vi "Format Attribute Value String.vi"(8 "error in (no error)":errorcluster, 11 "Data":variant) -> (0 "error out":errorcluster, 3 "Value as String":string)   [LabVIEW 2020, in "Linked Lists.lvlib" / "Linked List.lvclass"]
uses:
  <vilib>/gpm_packages/@cs/linked-list/Source/Linked List/Linked List/Linked List.lvclass
  <vilib>/gpm_packages/@cs/data-type-serializer/source/Data Type/Data Type.lvclass
  <vilib>/Utility/Data Type/NI_Data Type.lvlib
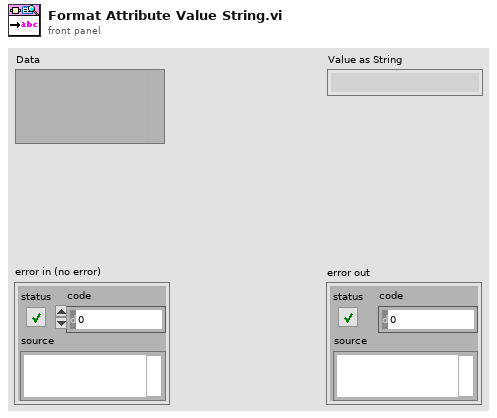
[diagram p1: front panel]
types:
  T1 = typedef "NI_Data Type.lvlib/Data Type.ctl" = enum8{"Invalid Type", "Void", "I8", "I16", "I32", "I64", "U8", "U16", "U32", "U64", "Single Float", "Double Float", "Extended Float", "Single Complex", "Double Complex", "Extended Complex", "Enum U8", "Enum U16", "Enum U32", "Enum U64", "Single Float With Unit", "Double Float With Unit", "Extended Float With Unit", "Single Complex with Unit", "Double Complex with Unit", "Extended Complex with Unit", "Boolean", "String", "Path", "Picture", "Tag", "Array", "Cluster", "Variant", "LV Variant", "Waveform", "Timestamp", "Digital Waveform", "Digital Data", "ExpressData", "Refnum", "External Data", "VI", "Poly VI", "LabVIEW Class Instance", "Fixed Point", "Set Collection", "Map Collection"}
  T2 = typedef "NI_Data Type.lvlib/Memory Info.ctl" = cluster{"Type":T3, "Size":u32}
  T3 = typedef "NI_Data Type.lvlib/Memory Type.ctl" = enum16{"Variable", "Fixed", "Bounded"}
  T4 = typedef "NI_Data Type.lvlib/Refnum Type.ctl" = enum16{"NotARefnum", "UnknownRefnum", "Generic", "Datalog", "ByteStream", "Device", "Occurence", "TCPNetConnection", "Auto", "Menu", "Imaq", "Hardware", "DataSocket", "Visa", "IVI", "UDPNetConnection", "Notifier", "Queue", "Irda", "EventReg", "DotNet", "UserEvent", "Callback", "UNUSED_EMPTY_POSITION", "BlueToothNetConnection", "LVObjApp", "LVObjVI", "LVObjUnknown", "GenericClass", "UserDefinedRefnumTag", "DataValue", "RT FIFO", "TDMS File", "PythonSessionRefnum"}
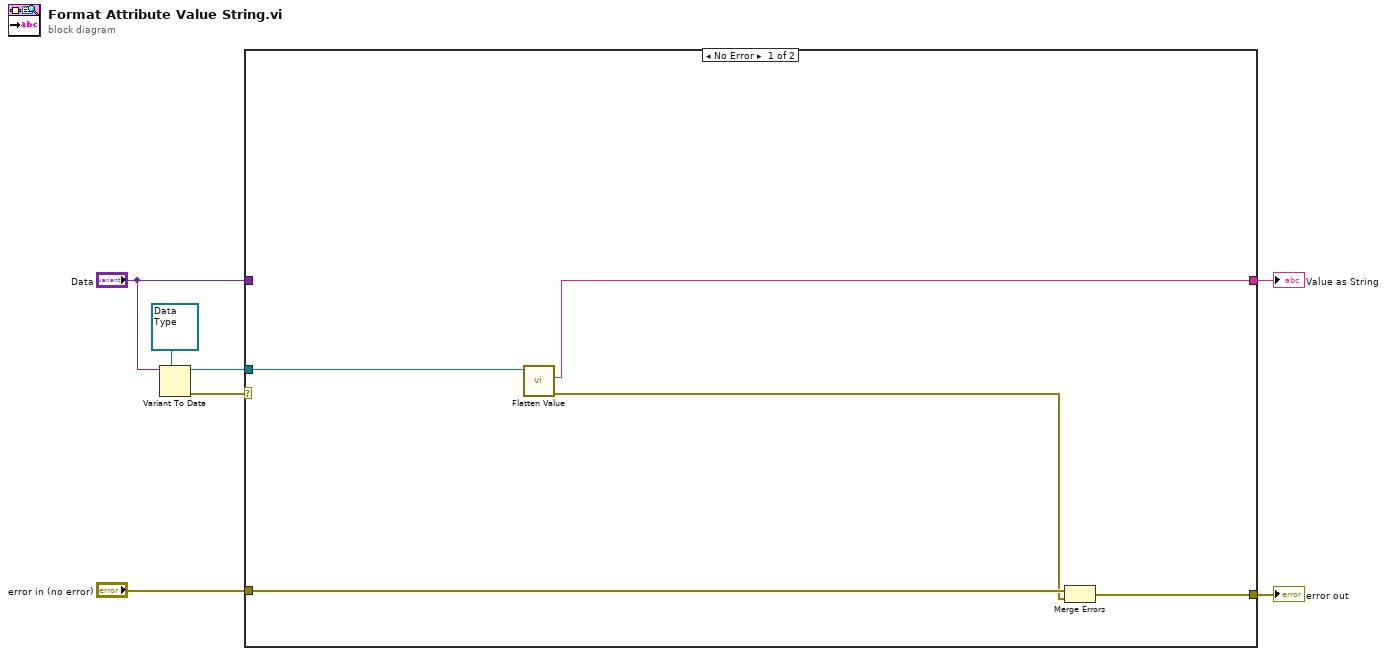
[diagram p0: block diagram]
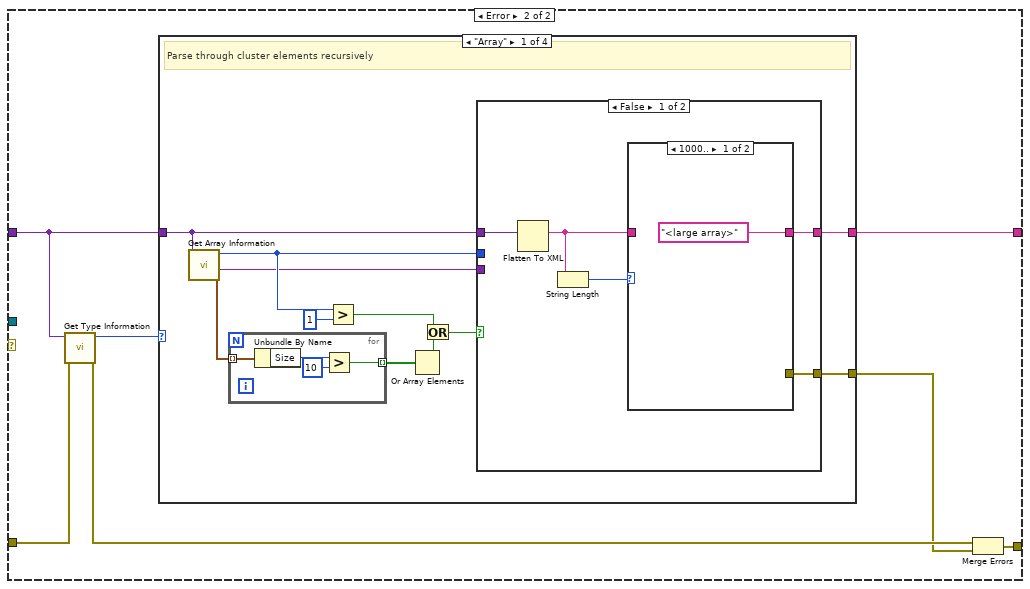
[diagram p2: hidden frame]
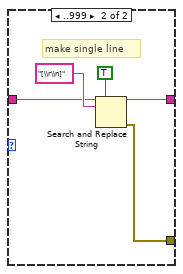
[diagram p3: hidden frame]
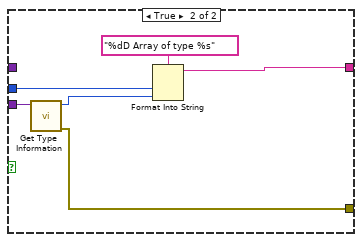
[diagram p4: hidden frame]
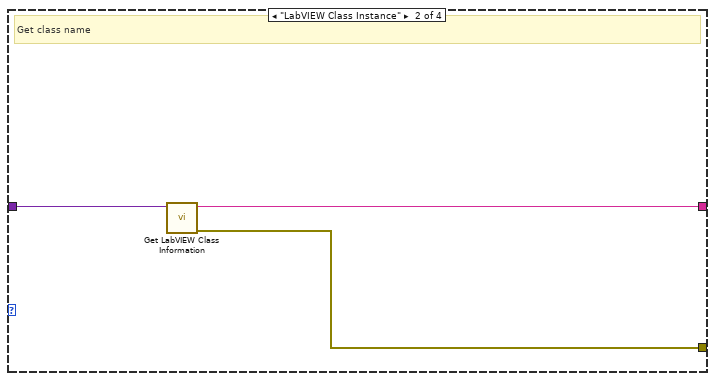
[diagram p5: hidden frame]
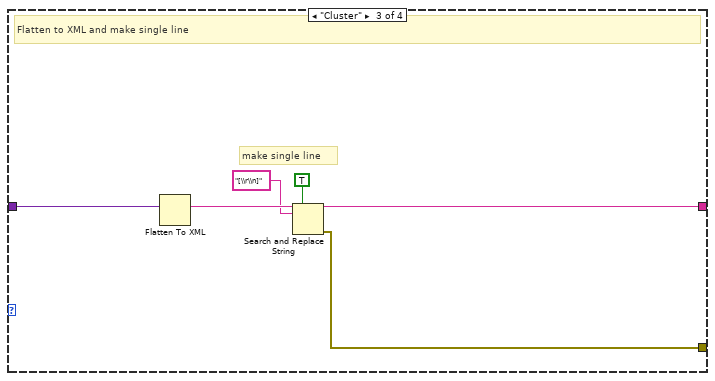
[diagram p6: hidden frame]
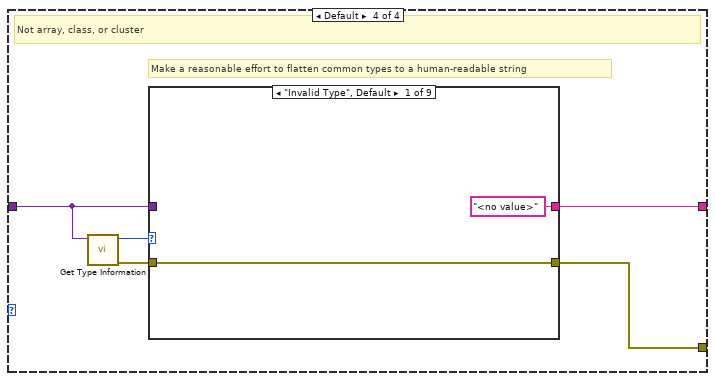
[diagram p7: hidden frame]
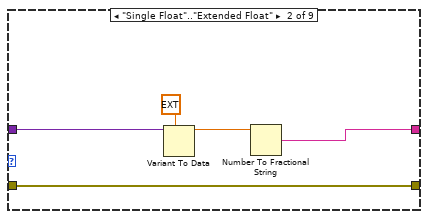
[diagram p8: hidden frame]
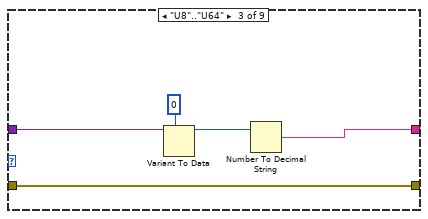
[diagram p9: hidden frame]
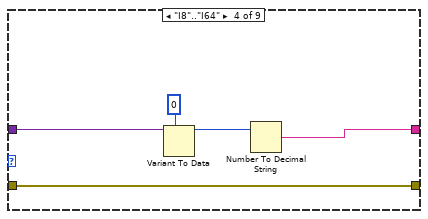
[diagram p10: hidden frame]
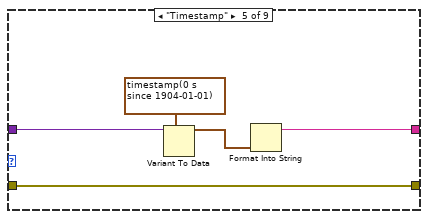
[diagram p11: hidden frame]
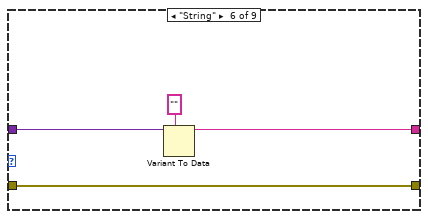
[diagram p12: hidden frame]
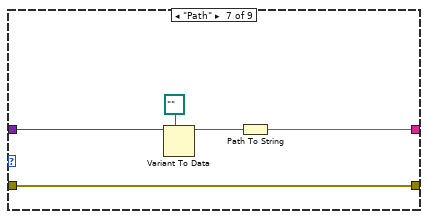
[diagram p13: hidden frame]
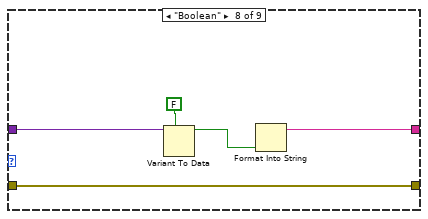
[diagram p14: hidden frame]
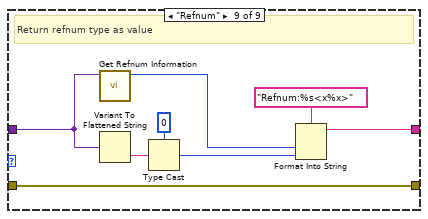
[diagram p15: hidden frame]
diagram:
  n1 = Variant To Data(type=refnum<class "Data Type.lvclass"> refnum ("Data Type.lvclass"), Variant="Data") -> (data=w1:refnum<class "Data Type.lvclass">, error out=w2:errorcluster)  [unwired: 1 in]
  n2 = case shown="No Error" w2 {
    tunnel: [w11 w19] -> w7
    tunnel: "error in (no error)" -> [w10 w16]
    tunnel: [w8 w15] -> w5
    tunnel: "Data" -> [_ w13]
    tunnel: w1 -> [w12 _]
    frame No Error {
      n3 = call-dynamic "Flatten Value.vi"("Data Type in"=w12) -> ("error out"=w9:errorcluster, "Value"=w11:string)  [unwired: 8 in, 1 out]
      n4 = Merge Errors(w10, w9) -> (w8:errorcluster)
    }
    frame Error {
      n5 = call <vilib>:"Get Type Information.vi"("error in (no error)"=w16, "variant"=w13) -> ("error out"=w17:errorcluster, "type"=w18:T1)  [unwired: 5 in, 3 out]
      n6 = case shown="\"Array\"" w18 {
        tunnel: [w30 w53 w60 w62] -> w19
        tunnel: w13 -> [w28 w54 w59 w63]
        tunnel: [w29 w52 w55 w61] -> w14
        frame "Array" {
          # "Parse through cluster elements recursively"
          n7 = call <vilib>:"Get Array Information.vi"("variant"=w28) -> ("array element data type"=w20:variant, "array lengths"=w21:T2[], "number of dimensions"=w22:i32)  [unwired: 7 in, 1 out]
          n8 = for {
            tunnel: w21 -> [w51] mode=indexing
            tunnel: [w48] -> w26 mode=indexing
            n9 = Unbundle By Name(w51) -> ("Size"=w50:u32)
            n10 = Greater?(x=w50, y=u32 10) -> (0:w48:bool)
          }
          n11 = Greater?(x=w22, y=1) -> (0:w24:bool)
          n12 = Or Array Elements(Boolean array=w26) -> (logical OR=w25:bool)
          n13 = Or(x=w24, y=w25) -> (x .or. y?=w23:bool)
          n14 = case shown="False" w23 {
            tunnel: [w35 w42] -> w30
            tunnel: [w34 w46] -> w29
            tunnel: w28 -> [w33 _]
            tunnel: w22 -> [_ w44]
            tunnel: w20 -> [_ w47]
            frame False {
              n15 = Flatten To XML(6:w33) -> (2:w32:string)
              n16 = String Length(string=w32) -> (length=w31:i32)
              n17 = case shown="1000.." w31 {
                tunnel: ["<large array>" w41] -> w35
                tunnel: [_ w38] -> w34
                tunnel: w32 -> [_ w37]
                frame 1000.. {
                }
                frame ..999 {
                  # "make single line"
                  n18 = Search and Replace String(replace all?=TRUE ("replace all? (F)"), input string=w37, search string="[\\r\\n]") -> (result string=w41:string, error out=w38:errorcluster)  [unwired: 5 in, 2 out]
                }
              }
            }
            frame True {
              n19 = call <vilib>:"Get Type Information.vi"("variant"=w47) -> ("error out"=w46:errorcluster, "type"=w43:T1)  [unwired: 6 in, 3 out]
              n20 = Format Into String(format string="%dD Array of type %s", w44, w43) -> (resulting string=w42:string)  [unwired: 2 in, 1 out]
            }
          }
        }
        frame "LabVIEW Class Instance" {
          # "Get class name"
          n21 = call <vilib>:"Get LabVIEW Class Information.vi"("variant"=w54) -> ("error out"=w52:errorcluster, "LabVIEW class file name"=w53:string)  [unwired: 8 in, 1 out]
        }
        frame "Cluster" {
          # "make single line"
          # "Flatten to XML and make single line"
          n22 = Flatten To XML(6:w59) -> (2:w58:string)
          n23 = Search and Replace String(replace all?=TRUE ("replace all? (F)"), input string=w58, search string="[\\r\\n]") -> (result string=w60:string, error out=w55:errorcluster)  [unwired: 5 in, 2 out]
        }
        frame Default {
          # "Make a reasonable effort to flatten common types to a human-readable string"
          # "Not array, class, or cluster"
          n24 = call <vilib>:"Get Type Information.vi"("variant"=w63) -> ("error out"=w65:errorcluster, "type"=w64:T1)  [unwired: 6 in, 3 out]
          n25 = case shown="\"Invalid Type\", Default" w64 {
            tunnel: w63 -> [_ w71 w76 w81 w86 w90 w95 w100 w105]
            tunnel: ["<no value>" w70 w75 w80 w83 w89 w93 w97 w107] -> w62
            tunnel: w65 -> [w67 w68 w73 w78 w85 w88 w92 w99 w109]
            tunnel: [w67 w68 w73 w78 w85 w88 w92 w99 w109] -> w61
            frame "Invalid Type", Default {
            }
            frame "Single Float".."Extended Float" {
              n26 = Variant To Data(type=ext 0.0, Variant=w71) -> (data=w69:ext)  [unwired: 1 in, 1 out]
              n27 = Number To Fractional String(number=w69) -> (F-format string=w70:string)  [unwired: 3 in]
            }
            frame "U8".."U64" {
              n28 = Variant To Data(type=u64 0, Variant=w76) -> (data=w74:u64)  [unwired: 1 in, 1 out]
              n29 = Number To Decimal String(number=w74) -> (decimal integer string=w75:string)  [unwired: 1 in]
            }
            frame "I8".."I64" {
              n30 = Variant To Data(type=i64 0, Variant=w81) -> (data=w79:i64)  [unwired: 1 in, 1 out]
              n31 = Number To Decimal String(number=w79) -> (decimal integer string=w80:string)  [unwired: 1 in]
            }
            frame "Timestamp" {
              n32 = Variant To Data(type=timestamp(0 s since 1904-01-01), Variant=w86) -> (data=w84:timestamp)  [unwired: 1 in, 1 out]
              n33 = Format Into String(w84) -> (resulting string=w83:string)  [unwired: 3 in, 1 out]
            }
            frame "String" {
              n34 = Variant To Data(type="", Variant=w90) -> (data=w89:string)  [unwired: 1 in, 1 out]
            }
            frame "Path" {
              n35 = Variant To Data(type=path "", Variant=w95) -> (data=w94:path)  [unwired: 1 in, 1 out]
              n36 = Path To String(path=w94) -> (string=w93:string)
            }
            frame "Boolean" {
              n37 = Variant To Data(type=FALSE, Variant=w100) -> (data=w98:bool)  [unwired: 1 in, 1 out]
              n38 = Format Into String(w98) -> (resulting string=w97:string)  [unwired: 3 in, 1 out]
            }
            frame "Refnum" {
              # "Return refnum type as value"
              n39 = call <vilib>:"Get Refnum Information.vi"("variant"=w105) -> ("reference type"=w108:T4)  [unwired: 7 in, 3 out]
              n40 = Variant To Flattened String(Variant=w105) -> (data string=w104:string)  [unwired: 1 out]
              n41 = Type Cast(type=u32 0, x=w104) -> (*(type *) &x=w102:u32)
              n42 = Format Into String(format string="Refnum:%s<x%x>", w108, w102) -> (resulting string=w107:string)  [unwired: 2 in, 1 out]
            }
          }
        }
      }
      n43 = Merge Errors(w17, w14) -> (w15:errorcluster)
    }
  }
  "error out" <- w5
  "Value as String" <- w7
